vi "AnalyDecayPhosphoAndSystem.vi"(0 "Scan rate (Hz)":dbl, 1 "Raw Data Image":T1, 5 "N pulses":i32=10, 9 "Skip samples":i32=12, 11 "Last samples":i32=5, 12 "N samples/decay":i32=150) -> (3 "mean and fit":dbl[][](graph), 4 "amplitude":dbl=1.3790672561842066 caption="Amplitude (au)" format="%#_3g", 6 "Tau (us)":dbl=8.774972224805227 format="%#_3g", 10 "Residu (au)":dbl=8.774972224805227 format="%#_3g", 13 "Standard error Amplitude":dbl=8.774972224805227 format="%#_3g", 14 "Standard error Tau (us)":dbl=8.774972224805227 format="%#_3g", 15 "Area (au)":dbl=8.774972224805227 format="%#_3g")   [LabVIEW 2013]
uses:
  <vilib>/vision/Image Controls.llb/IMAQ Image.ctl
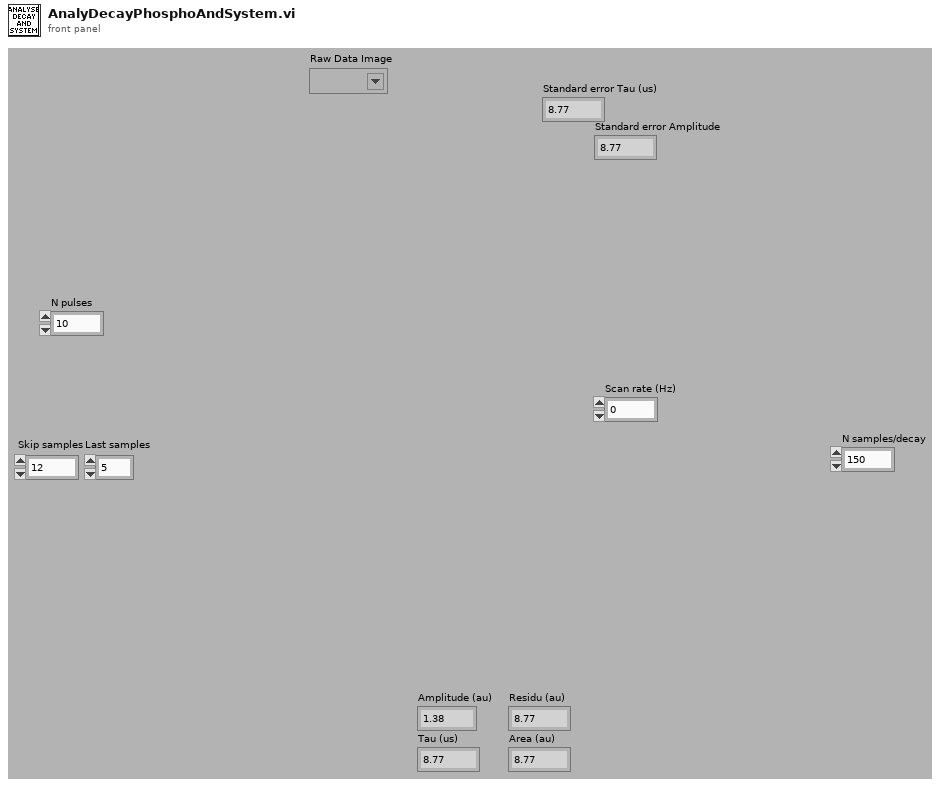
[diagram p1: front panel]
types:
  T1 = typedef "IMAQ Image.ctl" = refnum<image>
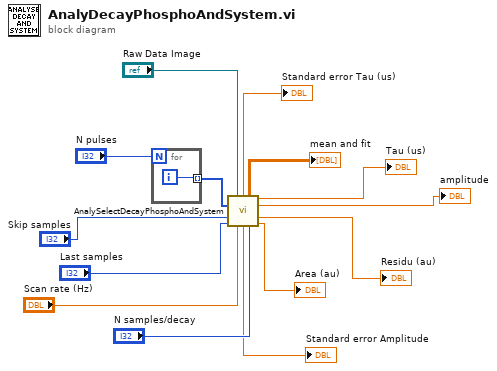
[diagram p0: block diagram]
diagram:
  n1 = for {
    N: "N pulses" -> [_]
    tunnel: [w15] -> w1 mode=indexing
    i -> [w15]
  }
  n2 = call "AnalySelectDecayPhosphoAndSystem.vi"("Raw Data Image"="Raw Data Image", "Pulses matrice"=w1, "Skip samples"="Skip samples", "Last samples"="Last samples", "Scan rate (Hz)"="Scan rate (Hz)", "N samples/decay"="N samples/decay") -> ("Standard error Tau (us)"=→"Standard error Tau (us)":dbl, "mean and fit"=→"mean and fit":dbl[][], "Tau (us)"=→"Tau (us)":dbl, "amplitude"=→"amplitude":dbl, "Residu (au)"=→"Residu (au)":dbl, "Standard error Amplitude"=→"Standard error Amplitude":dbl, "Area (au)"=→"Area (au)":dbl)  [unwired: 3 in]
